vi "IMAQdx Sequence2.vi"(7 "Timeout (ms)":i32=5000, 8 "error in":errorcluster, 10 "Images In":T1[](array[typedef]), 11 "Session In":T2) -> (0 "error out":errorcluster, 2 "Images Out":T1[](array[typedef]), 3 "Session Out":T2)   [LabVIEW 2020, in "NI_Vision_Acquisition_Software.lvlib"]
doc: "Configures, starts, acquires, stops, and unconfigures a sequence acquisition. Use this VI to capture multiple images. If you call this VI before calling the IMAQdx Open Camera VI, the IMAQdx Sequence2 VI uses cam0 by default."
uses:
  NI_Vision_Acquisition_Software.lvlib
  IMAQdx.ctl
  IMAQ Image.ctl
  IMAQdx Acquisition Mode.ctl
  IMAQdx Buffer Number Mode.ctl
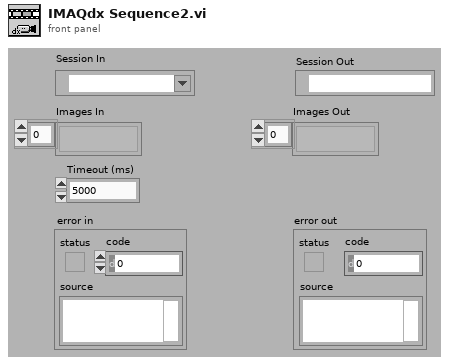
[diagram p1: front panel]
types:
  T1 = typedef "IMAQ Image.ctl" = refnum<image>
  T2 = typedef "IMAQdx.ctl" = refnum<k21>
  T3 = typedef "NI_Vision_Acquisition_Software.lvlib/IMAQdx Buffer Number Mode.ctl" = enum32{"Next", "Last", "Buffer Number", "Every", "Last New"}
  T4 = typedef "NI_Vision_Acquisition_Software.lvlib/IMAQdx Acquisition Mode.ctl" = enum32{"One Shot", "Continuous"}
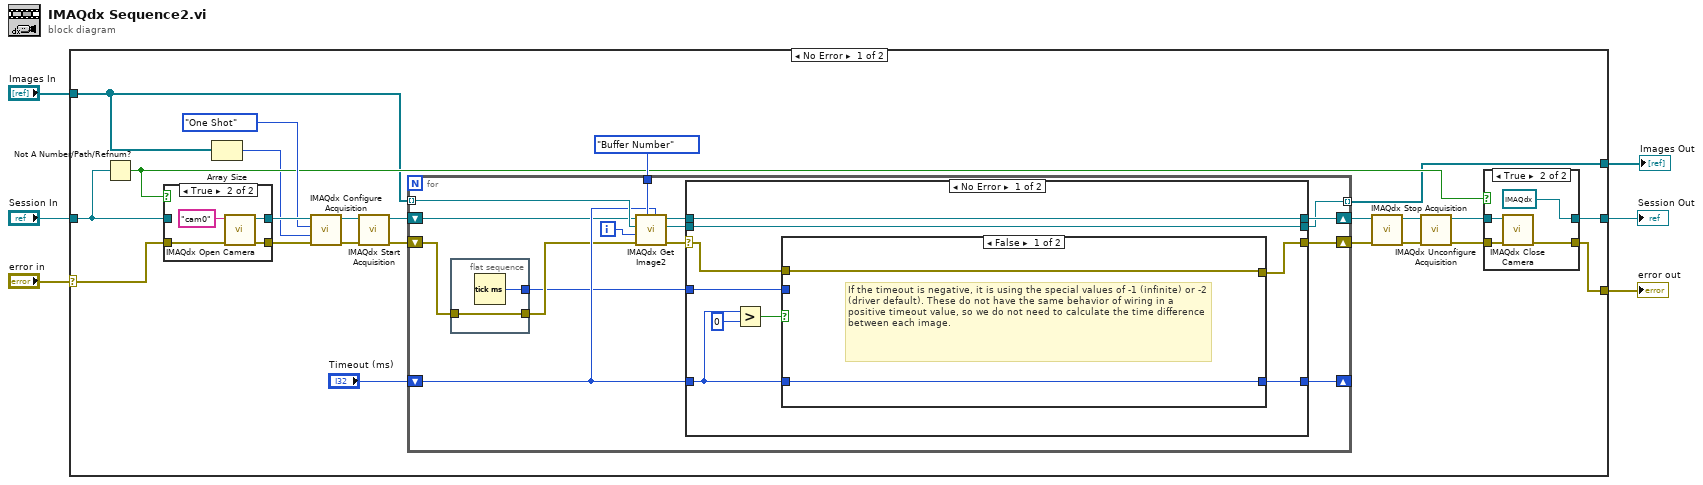
[diagram p0: block diagram]
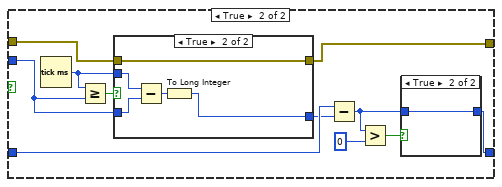
[diagram p2: hidden frame]
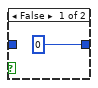
[diagram p3: hidden frame]
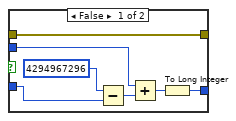
[diagram p4: hidden frame]
diagram:
  n1 = case shown="No Error" "error in" {
    selector: "error in" -> [w7 w101]
    tunnel: "Session In" -> [w28 w100]
    tunnel: [w15 w100] -> w5
    tunnel: [w14 w101] -> w4
    tunnel: "Images In" -> [w12 w99]
    tunnel: [w11 w99] -> w2
    frame No Error {
      n2 = Not A Number/Path/Refnum?(number/path/refnum=w28) -> (NaN/Path/Refnum?=w16:bool)
      n3 = case shown="True" w16 {
        tunnel: [w94 w98] -> w29
        tunnel: w28 -> [w94 _]
        tunnel: [w93 w97] -> w27
        tunnel: w7 -> [w93 w96]
        frame False {
        }
        frame True {
          n4 = call "IMAQdx Open Camera.vi"("error in"=w96, "Session In"="cam0") -> ("error out"=w97:errorcluster, "Session Out"=w98:T2)  [unwired: 8 in]
        }
      }
      n5 = Array Size(array=w12) -> (size(s)=w13:i32)
      n6 = call "IMAQdx Configure Acquisition.vi"("error in"=w27, "Number of Buffers"=w13, "Continuous?"=IMAQdx_Acquisition_Mode."One Shot", "Session In"=w29) -> ("error out"=w24:errorcluster, "Session Out"=w25:T2)  [unwired: 6 in]
      n7 = call "IMAQdx Start Acquisition.vi"("error in"=w24, "Session In"=w25) -> ("error out"=w9:errorcluster, "Session Out"=w10:T2)  [unwired: 8 in]
      n8 = for {
        tunnel: IMAQdx_Buffer_Number_Mode."Buffer Number" ("Buffer Number Mode") -> [w44]
        shift-right: [w40] -> w21
        shift-left: w9 -> [w33]
        shift-right: [w38] -> w22
        shift-left: w10 -> [w32]
        tunnel: w12 -> [w42] mode=indexing
        tunnel: [w36] -> w11 mode=indexing
        shift-right: [w35] -> _
        shift-left: "Timeout (ms)" -> [w34]
        i -> [w43]
        n9 = flat-sequence {
          tunnel: w33 -> [w46]
          tunnel: [w46] -> w31
          tunnel: [w45] -> w30
          frame #0 {
            n10 = Tick Count (ms)() -> (millisecond timer value=w45:u32)
          }
        }
        n11 = call "IMAQdx Get Image2.vi"("Timeout (ms)"=w34, "Buffer Number Mode (Next)"=w44, "error in"=w31, "Buffer Number In"=w43, "Image In"=w42, "Session In"=w32) -> ("error out"=w41:errorcluster, "Image Out"=w37:T1, "Session Out"=w39:T2)  [unwired: 2 in, 1 out]
        n12 = case shown="No Error" w41 {
          selector: w41 -> [w50 w86]
          tunnel: [w52 w86] -> w40
          tunnel: w39 -> [w55 w85]
          tunnel: [w55 w85] -> w38
          tunnel: [w54 w84] -> w36
          tunnel: w37 -> [w54 w84]
          tunnel: w30 -> [w53 _]
          tunnel: w34 -> [w48 w83]
          tunnel: [w51 w83] -> w35
          frame No Error {
            n13 = Greater?(x=w48, y=0) -> (0:w49:bool)
            n14 = case shown="False" w49 {
              tunnel: w53 -> [_ w66]
              tunnel: [w57 w65] -> w52
              tunnel: w48 -> [w56 w61]
              tunnel: [w56 w59] -> w51
              tunnel: w50 -> [w57 w58]
              frame False {
                # "If the timeout is negative, it is using the special values of -1 (infinite) or -2 (driver default). These do not have the same behavior of wiring in a positive timeout value, so we do not need to calculate the time difference between each image."
              }
              frame True {
                n15 = Tick Count (ms)() -> (millisecond timer value=w67:u32)
                n16 = Greater Or Equal?(x=w67, y=w66) -> (x >= y?=w68:bool)
                n17 = case shown="True" w68 {
                  tunnel: w67 -> [w73 w81]
                  tunnel: w66 -> [w76 w82]
                  tunnel: w58 -> [w77 w79]
                  tunnel: [w77 w79] -> w65
                  tunnel: [w72 w78] -> w60
                  frame False {
                    n18 = Subtract(x=u64 4294967296, y=w76) -> (x-y=w74:u64)
                    n19 = Add(x=w73, y=w74) -> (x+y=w71:u64)
                    n20 = To Long Integer(number=w71) -> (32bit integer=w72:i32)
                  }
                  frame True {
                    n21 = Subtract(x=w81, y=w82) -> (x-y=w80:u32)
                    n22 = To Long Integer(number=w80) -> (32bit integer=w78:i32)
                  }
                }
                n23 = Subtract(x=w61, y=w60) -> (x-y=w62:i32)
                n24 = Greater?(x=w62, y=0) -> (0:w63:bool)
                n25 = case shown="True" w63 {
                  tunnel: w62 -> [_ w70]
                  tunnel: [0 w70] -> w59
                  frame False {
                  }
                  frame True {
                  }
                }
              }
            }
          }
          frame Error {
          }
        }
      }
      n26 = call "IMAQdx Stop Acquisition.vi"("error in"=w21, "Session In"=w22) -> ("error out"=w19:errorcluster, "Session Out"=w20:T2)  [unwired: 8 in]
      n27 = call "IMAQdx Unconfigure Acquisition.vi"("error in"=w19, "Session In"=w20) -> ("error out"=w18:errorcluster, "Session Out"=w17:T2)  [unwired: 8 in]
      n28 = case shown="True" w16 {
        tunnel: w18 -> [w87 w92]
        tunnel: w17 -> [w88 w90]
        tunnel: [w88 T2 refnum ("Session Out")] -> w15
        tunnel: [w87 w91] -> w14
        frame False {
        }
        frame True {
          n29 = call "IMAQdx Close Camera.vi"("error in"=w92, "Session In"=w90) -> ("error out"=w91:errorcluster)  [unwired: 9 in]
        }
      }
    }
    frame Error {
    }
  }
  "Session Out" <- w5
  "error out" <- w4
  "Images Out" <- w2
